vi "Reshape U16 Array.vi"(8 "error in (no error)":errorcluster, 10 "FrameDescription":T1, 11 "U16 Array":u16[](array[numeric])) -> (0 "error out":errorcluster, 3 "2D Array":u16[][](array[numeric]))   [LabVIEW 2014]
uses:
  controls/FrameDescription.ctl
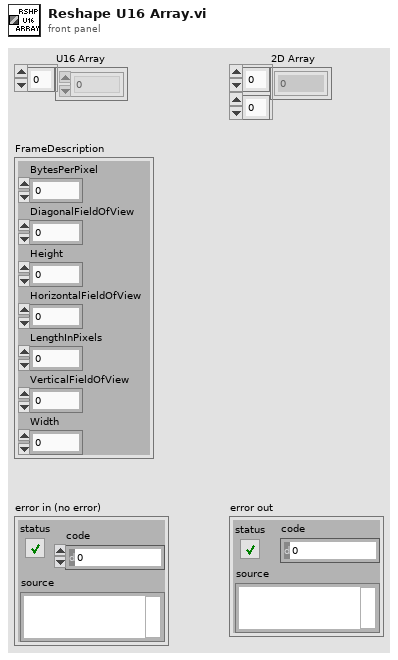
[diagram p1: front panel]
types:
  T1 = typedef "FrameDescription.ctl" = cluster{"BytesPerPixel":u32, "DiagonalFieldOfView":sgl, "Height":i32, "HorizontalFieldOfView":sgl, "LengthInPixels":u32, "VerticalFieldOfView":sgl, "Width":i32}
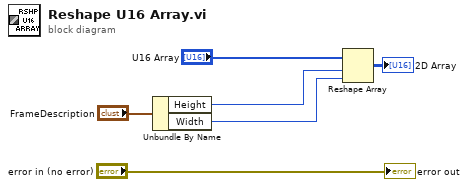
[diagram p0: block diagram]
diagram:
  n1 = Unbundle By Name("FrameDescription") -> ("Height"=w5:i32, "Width"=w4:i32)
  n2 = Reshape Array("U16 Array", w5, w4) -> (→"2D Array":u16[][])
  "error out" <- "error in (no error)"
